vi "LVFunction_Pupil draw Legendre Zernike.vi"(0 "TypePhase":T7=enum."Modal_Legendre", 2 "Cursor Position":T1, 5 "For Zernike":T9={"nb point"=180, "CircularProjectionPupilDimensions"={"Pupil center_sspp"={"X"=0.0, "Y"=0.0}, "Pupil radius_sspp"=0.0}}, 7 "RectangularProjectionPupilDimensions":T6, 9 "Commun 2":T5={"M13_Pupil"=refnum, "Dimensions_µm"={"Size"={"X"=200, "Y"=200}, "Step"={"X"=1.0, "Y"=1.0}}, "XYGraph Refnum"=refnum, "Plot Area:Size"={"Width"=64, "Height"=64}, "Plot Area:Position"={"Left"=64, "Top"=64}}) -> ()   [LabVIEW 2018]
uses:
  Controls/ZernikeProjectionPupilSetup.ctl
  Controls/Point2Df.ctl
  Controls/WavefrontReconstructionMode.ctl
  Controls/LegendreProjectionPupilSetup.ctl
  Controls/General dimensions definition.ctl
  Controls/Point2D.ctl
  <vilib>/Utility/miscctls.llb/LVPointDoubleTypeDef.ctl
panel:
  out "Cursor.Cursor Name":string
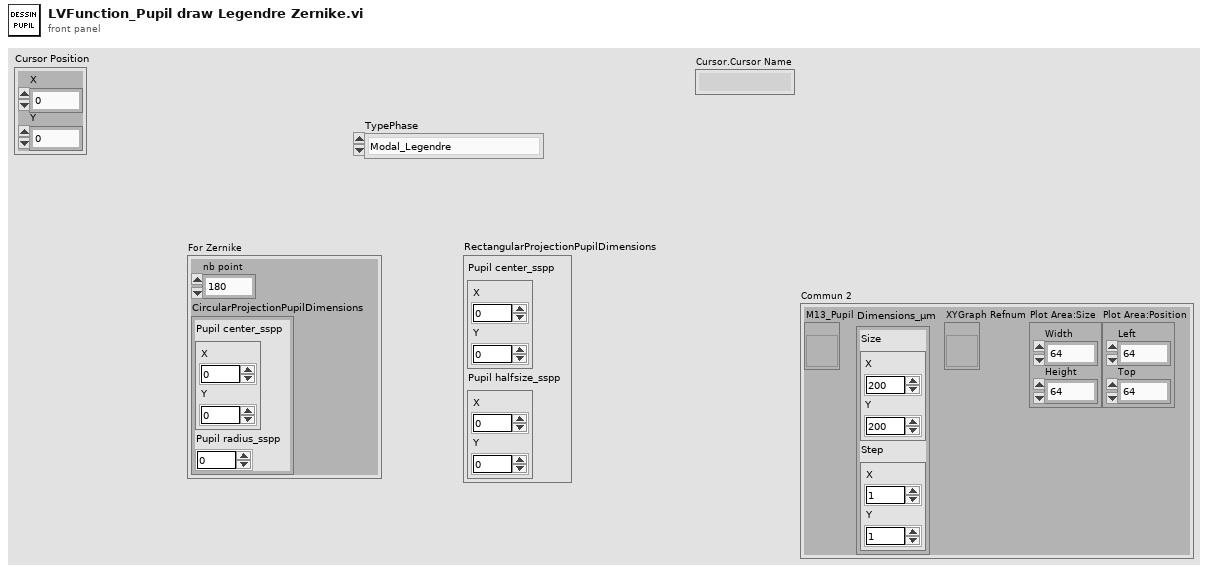
[diagram p1: front panel]
types:
  T1 = typedef "LVPointDoubleTypeDef.ctl" = cluster{"X":dbl, "Y":dbl}
  T2 = typedef "General dimensions definition.ctl" = cluster{"Size":T3, "Step":T4}
  T3 = typedef "Point2D.ctl" = cluster{"X":u32, "Y":u32}
  T4 = typedef "Point2Df.ctl" = cluster{"X":sgl, "Y":sgl}
  T5 = cluster{"M13_Pupil":refnum<vi>, "Dimensions_µm":T2, "XYGraph Refnum":refnum<vi>, "Plot Area:Size":cluster{"Width":u32, "Height":u32}, "Plot Area:Position":cluster{"Left":u32, "Top":u32}}
  T6 = typedef "LegendreProjectionPupilSetup.ctl" = cluster{"Pupil center_sspp":T4, "Pupil halfsize_sspp":T4}
  T7 = typedef "WavefrontReconstructionMode.ctl" = enum16{"None", "Modal_Legendre", "Modal_Zernike", "Zonal", "Modal_Zonal_Zernike", "Modal_Zonal_Legendre"}
  T8 = typedef "ZernikeProjectionPupilSetup.ctl" = cluster{"Pupil center_sspp":T4, "Pupil radius_sspp":sgl}
  T9 = cluster{"nb point":i32, "CircularProjectionPupilDimensions":T8}
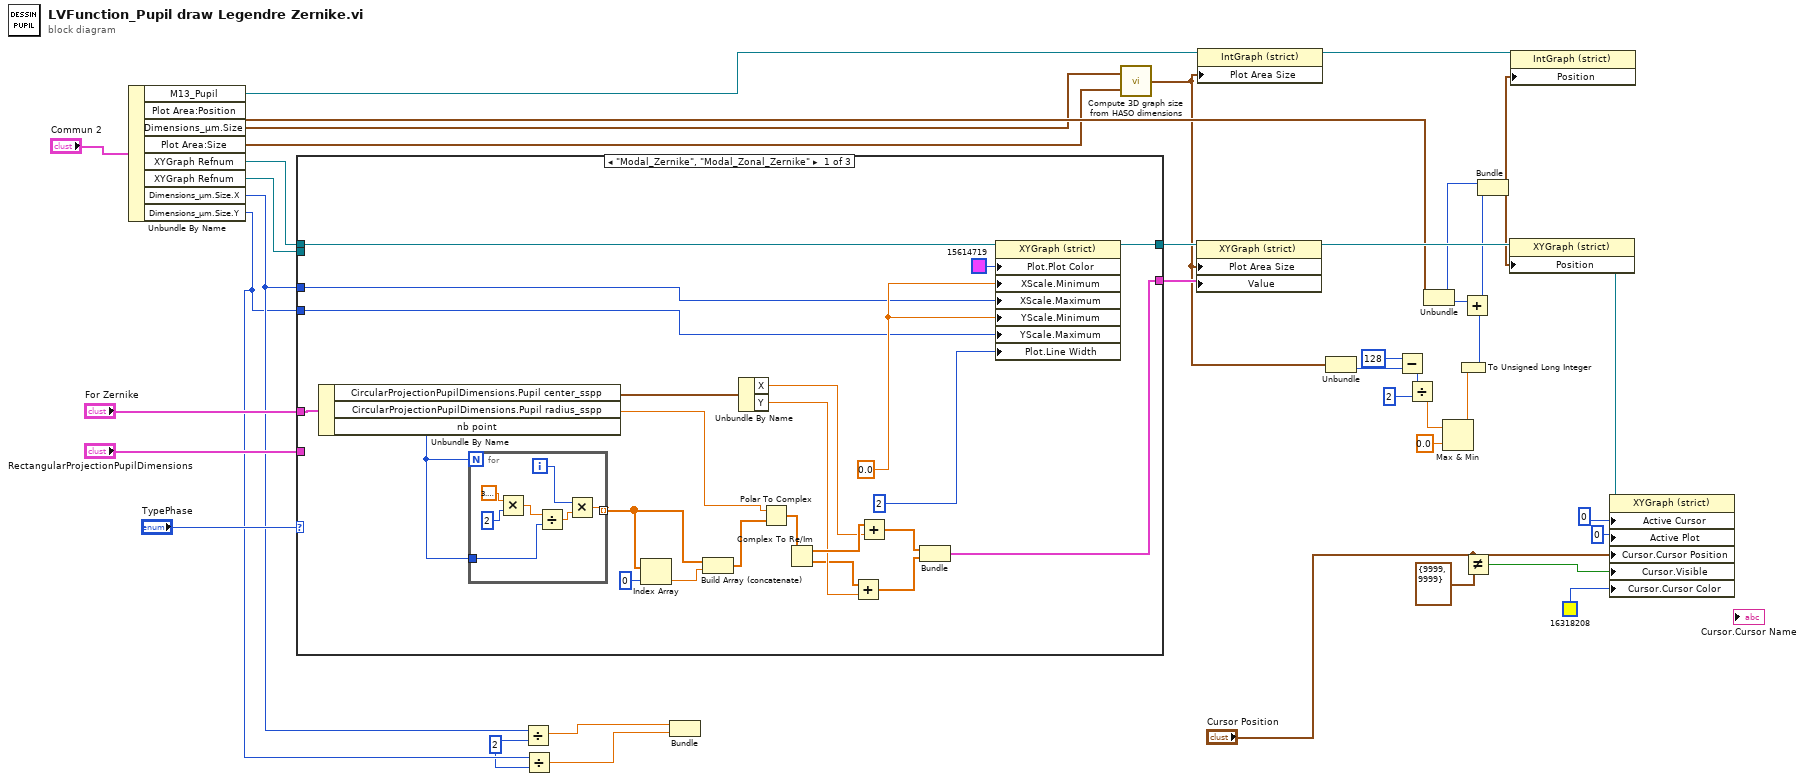
[diagram p0: block diagram]
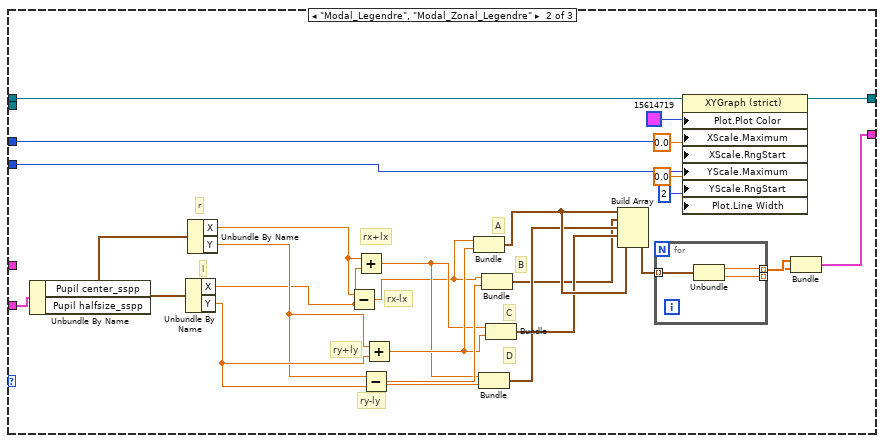
[diagram p2: hidden frame]
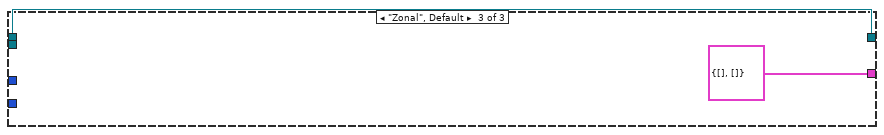
[diagram p3: hidden frame]
diagram:
  w11 = 2 ("index")
  n1 = Unbundle By Name("Commun 2") -> ("M13_Pupil"=w35:refnum<vi>, "Plot Area:Position"=w21:cluster{"Left":u32, "Top":u32}, "Dimensions_µm.Size"=w3:T3, "Plot Area:Size"=w2:cluster{"Width":u32, "Height":u32}, "XYGraph Refnum"=w31:refnum<vi>, "XYGraph Refnum"=w32:refnum<vi>, "Dimensions_µm.Size.X"=w15:u32, "Dimensions_µm.Size.Y"=w13:u32)
  n2 = case shown="\"Modal_Zernike\", \"Modal_Zonal_Zernike\"" "TypePhase" {
    tunnel: "For Zernike" -> [w50 _ _]
    tunnel: "RectangularProjectionPupilDimensions" -> [_ w80 _]
    tunnel: [w42 w72 cluster{dbl[], dbl[]} {[], []} ("Value")] -> w34
    tunnel: w31 -> [w46 w75 w100]
    tunnel: [w45 w74 w100] -> w33
    tunnel: w15 -> [w44 w70 _]
    tunnel: w13 -> [w43 w73 _]
    tunnel: w32 -> [_ _ _]
    frame "Modal_Zernike", "Modal_Zonal_Zernike" {
      w56 = 0.0 ("Y Scale.Range:Start")
      n3 = Unbundle By Name(w50) -> ("CircularProjectionPupilDimensions.Pupil center_sspp"=w41:T4, "CircularProjectionPupilDimensions.Pupil radius_sspp"=w49:sgl, "nb point"=w40:i32)
      n4 = for {
        N: w40 -> [_]
        tunnel: [w64] -> w59 mode=indexing
        tunnel: w40 -> [w63]
        i -> [w65]
        n5 = Multiply(x=3.141592653589793, y=2) -> (x*y=w67:dbl)
        n6 = Divide(x=w67, y=w63) -> (x/y=w66:dbl)
        n7 = Multiply(x=w65, y=w66) -> (x*y=w64:dbl)
      }
      n8 = Index Array(array=w59, index=0) -> (element=w58:dbl)
      n9 = Build Array (concatenate)(w59, w58) -> (w57:dbl[])
      n10 = Unbundle By Name(w41) -> ("X"=w54:sgl, "Y"=w53:sgl)
      n11 = Polar To Complex(1:w57, 2:w49) -> (0:w61:cdb[])
      n12 = Complex To Re/Im(x + iy=w61) -> (x=w55:dbl[], y=w52:dbl[])
      n13 = Add(x=w52, y=w53) -> (x+y=w47:dbl[])
      n14 = Add(x=w55, y=w54) -> (x+y=w48:dbl[])
      n15 = Bundle(w48, w47) -> (w42:cluster{dbl[], dbl[]})  [unwired: 1 in]
      n16 = property on="Property Node" class="XYGraph (strict)"(reference=w46, "Plot.Plot Color"=u32 15614719, "XScale.Minimum"=w56, "XScale.Maximum"=w44, "YScale.Minimum"=w56, "YScale.Maximum"=w43, "Plot.Line Width"=u8 2) -> (reference out=w45:refnum<vi>)  [unwired: 1 in, 1 out]
    }
    frame "Modal_Legendre", "Modal_Zonal_Legendre" {
      # "D"
      # "C"
      # "B"
      # "A"
      # "l"
      # "r"
      # "ry+ly"
      # "ry-ly"
      # "rx+lx"
      # "rx-lx"
      n17 = Unbundle By Name(w80) -> ("Pupil center_sspp"=w71:T4, "Pupil halfsize_sspp"=w79:T4)
      n18 = Unbundle By Name(w79) -> ("X"=w83:sgl, "Y"=w85:sgl)
      n19 = Unbundle By Name(w71) -> ("X"=w82:sgl, "Y"=w84:sgl)
      n20 = Subtract(x=w82, y=w83) -> (x-y=w86:sgl)
      n21 = Add(x=w82, y=w83) -> (x+y=w87:sgl)
      n22 = Subtract(x=w84, y=w85) -> (x-y=w89:sgl)
      n23 = Add(x=w84, y=w85) -> (x+y=w88:sgl)
      n24 = Bundle(w86, w88) -> (w93:cluster{sgl, sgl})  [unwired: 1 in]
      n25 = Bundle(w87, w89) -> (w91:cluster{sgl, sgl})  [unwired: 1 in]
      n26 = Bundle(w86, w89) -> (w90:cluster{sgl, sgl})  [unwired: 1 in]
      n27 = Bundle(w87, w88) -> (w92:cluster{sgl, sgl})  [unwired: 1 in]
      n28 = Build Array(w93, w90, w91, w92, w93) -> (w76:cluster{sgl, sgl}[])
      n29 = for {
        tunnel: w76 -> [w99] mode=indexing
        tunnel: [w98] -> w78 mode=indexing
        tunnel: [w97] -> w77 mode=indexing
        n30 = Unbundle(w99) -> (w98:sgl, w97:sgl)
      }
      n31 = property on="Property Node" class="XYGraph (strict)"(reference=w75, "Plot.Plot Color"=u32 15614719, "XScale.Maximum"=w70, "XScale.RngStart"=0.0 ("X Scale.Range:Minimum"), "YScale.Maximum"=w73, "YScale.RngStart"=0.0 ("Y Scale.Range:Minimum"), "Plot.Line Width"=u8 2) -> (reference out=w74:refnum<vi>)  [unwired: 1 in, 1 out]
      n32 = Bundle(w78, w77) -> (w72:cluster{sgl[], sgl[]})  [unwired: 1 in]
    }
    frame "Zonal", Default {
    }
  }
  n33 = Divide(x=w15, y=w11) -> (x/y=w14:dbl)
  n34 = Divide(x=w13, y=w11) -> (x/y=w12:dbl)
  n35 = Bundle(w14, w12) -> ()  [unwired: 1 in, 1 out]
  n36 = call "Compute 3D graph size from HASO dimensions.vi"("Plot Area:Size 2"=w2, "Size"=w3) -> ("Plot Area:Size"=w1:cluster{"Width":u32, "Height":u32})
  n37 = property on="Property Node" class="XYGraph (strict)"(reference=w33, "Plot Area Size"=w1, "Value"=w34) -> (reference out=w29:refnum<vi>)  [unwired: 1 in, 1 out]
  n38 = property on="Property Node" class="IntGraph (strict)"(reference=w35, "Plot Area Size"=w1) -> (reference out=w30:refnum<vi>)  [unwired: 1 in, 1 out]
  n39 = Unbundle(w1) -> ("Height"=w28:u32)  [unwired: 1 out]
  n40 = Subtract(x=u32 128, y=w28) -> (x-y=w26:u32)
  n41 = Divide(x=w26, y=u32 2) -> (x/y=w18:dbl)
  n42 = Unbundle(w21) -> ("Left"=w23:u32, "Top"=w24:u32)
  n43 = Max & Min(x=w18, y=sgl 0.0) -> (max(x,y)=w17:dbl)  [unwired: 1 out]
  n44 = To Unsigned Long Integer(number=w17) -> (unsigned 32bit integer=w16:u32)
  n45 = Add(x=w24, y=w16) -> (x+y=w22:u32)
  n46 = Not Equal?(x="Cursor Position", y=T3 {"X"=9999, "Y"=9999} ("StartSubPupilFromHasoData")) -> (x != y?=w8:bool)
  n47 = Bundle("Left"=w23, w22) -> (w20:cluster{"Left":u32, u32})  [unwired: 1 in]
  n48 = property on="Property Node" class="XYGraph (strict)"(reference=w29, "Position"=w20) -> (reference out=w10:refnum<vi>)  [unwired: 1 in, 1 out]
  n49 = property on="Property Node" class="IntGraph (strict)"(reference=w30, "Position"=w20) -> ()  [unwired: 1 in, 2 out]
  n50 = property on="Property Node" class="XYGraph (strict)"(reference=w10, "Active Cursor"=u32 0, "Active Plot"=u32 0, "Cursor.Cursor Position"="Cursor Position", "Cursor.Visible"=w8, "Cursor.Cursor Color"=u32 16318208) -> ()  [unwired: 1 in, 2 out]
